vi "Get Next.vi"(0 "Subroutine in":refnum<class "Subroutine.lvclass">, 1 "Linked List Ref":refnum<data-value>, 5 "Active Unique ID":string, 9 "Active Element Index":i32, 11 "error in (no error)":errorcluster) -> (3 "Linked List Ref out":refnum<data-value>, 4 "Executioner out":refnum<class "Executioner.lvclass">, 6 "Active Unique ID out":string, 8 "Test Executive Ref out":refnum<data-value>, 10 "Active Element Index out":i32, 12 "Found":bool, 13 "Complete":bool, 14 "Stop":bool, 15 "error out":errorcluster)   [LabVIEW 2019, in "Test Executive.lvlib" / "Subroutine.lvclass"]
uses:
  <vilib>/gpm_packages/@cs/test-executive/Source/Test Executive/Subroutine/Subroutine.lvclass
  C:/Program Files/National Instruments/LabVIEW 2019/vi.lib/gpm_packages/@cs/test-executive/Source/Test Executive/Executioner/Executioner.lvclass
  <vilib>/gpm_packages/@cs/test-executive/Source/Test Executive/Executioner/Executioner.lvclass
  <vilib>/gpm_packages/@cs/linked-list/Source/Linked List/ILinkedList/ILinked List.lvclass
  <vilib>/gpm_packages/@cs/test-executive/Source/Test Executive/ITestExecutive/ITest Executive.lvclass
  28e86f38-66cc-4303-ad50-260c1a8a0bf4.vi
  bb82cf1c-3602-4c17-aaf6-92fbf2a690c8.vi
  2b196b4b-1a84-4c76-b20a-ced8a0baa885.vi
  296adc96-2638-4d5e-ba7f-24ec80cc44f5.vi
  bf42a184-1053-416f-aa66-ef3d33315e6b.vi
  c3880502-fd26-4328-86fb-66246f65a8d7.vi
  <vilib>/Utility/error.llb/Error Cluster From Error Code.vi
  <vilib>/gpm_packages/@cs/linked-list/Source/Linked List/Linked List Ref/Linked List Ref.lvclass
  <vilib>/gpm_packages/@cs/test-executive/Source/Test Executive/TestExecutive Ref/TestExecutive Ref.lvclass
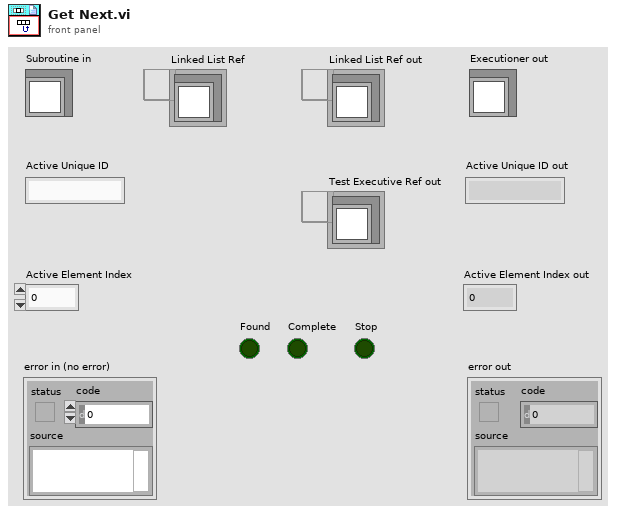
[diagram p1: front panel]
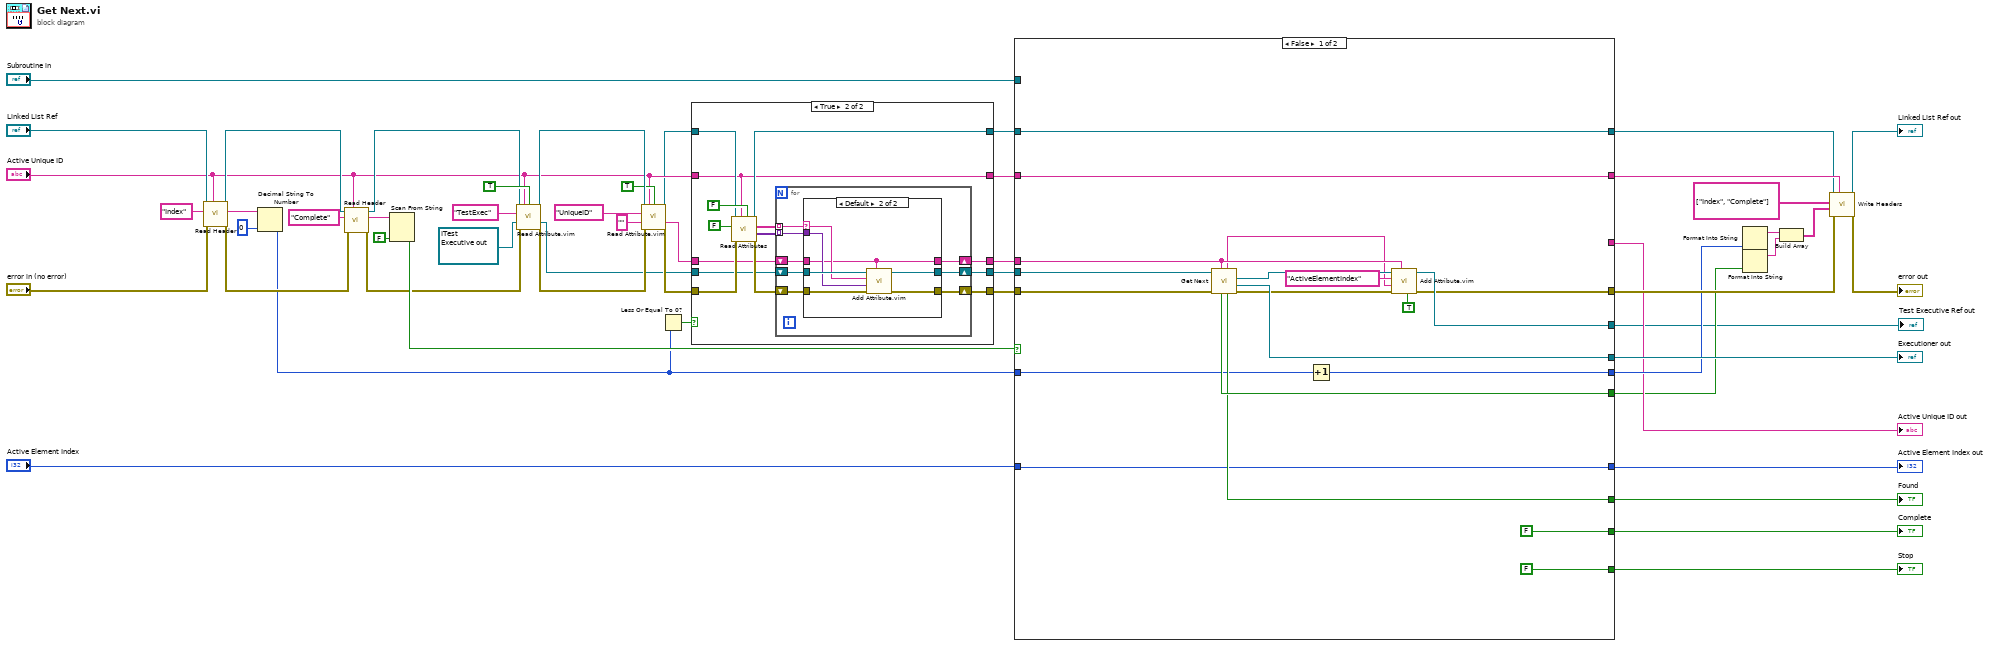
[diagram p0: block diagram]
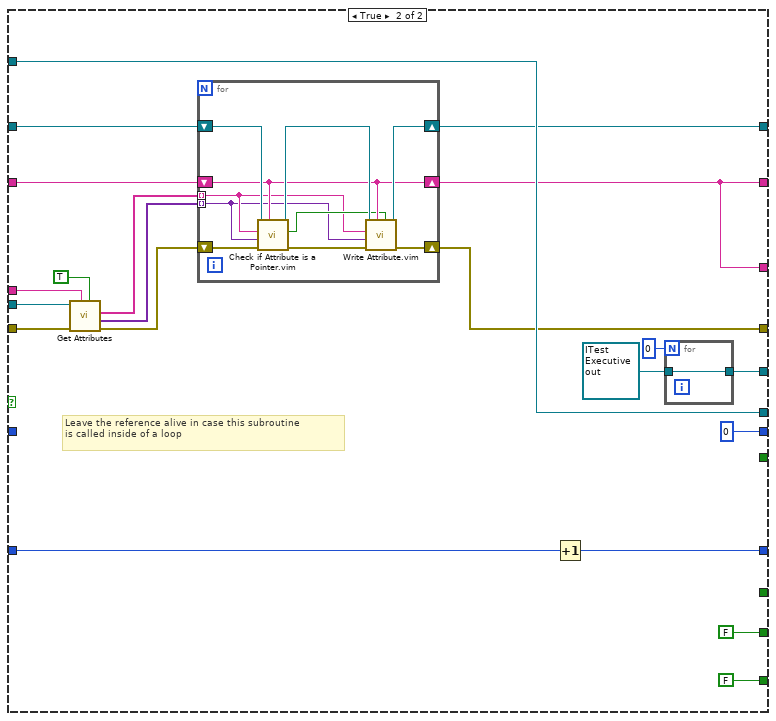
[diagram p4: hidden frame]
diagram:
  n1 = call <vilib>:"Read Header.vi"("Linked List ID"="Active Unique ID", "error in (no error)"="error in (no error)", "Header Name"="Index" ("Attribute Name"), "Linked List Ref"="Linked List Ref") -> ("error out"=w30:errorcluster, "Header Value"=w36:string, "Linked List Ref out"=w31:refnum<data-value>)  [unwired: 4 in, 1 out]
  n2 = Decimal String To Number(string=w36, default (0L)=0 ("Attribute")) -> (number=w1:i32)  [unwired: 1 in, 1 out]
  n3 = call <vilib>:"Read Header.vi"("Linked List ID"="Active Unique ID", "error in (no error)"=w30, "Header Name"="Complete" ("Attribute Name"), "Linked List Ref"=w31) -> ("error out"=w13:errorcluster, "Header Value"=w33:string, "Linked List Ref out"=w14:refnum<data-value>)  [unwired: 4 in, 1 out]
  n4 = Scan From String(input string=w33, default 1=FALSE) -> (output 1=w38:bool)  [unwired: 3 in, 3 out]
  n5 = call "Read Attribute.vim"("Linked List Ref"=w14, "Linked List ID"="Active Unique ID", "Include Private?"=TRUE, "Attribute Name"="TestExec", "Type"=refnum<data-value> refnum ("Test Executive Ref out"), "error in (no error)"=w13) -> ("Linked List Ref out"=w19:refnum<data-value>, "Attribute"=w7:refnum<data-value>, "error out"=w17:errorcluster)  [unwired: 4 in, 3 out]
  n6 = call "Read Attribute.vim"("Linked List Ref"=w19, "Linked List ID"="Active Unique ID", "Include Private?"=TRUE, "Attribute Name"="UniqueID", "Type"="", "error in (no error)"=w17) -> ("Linked List Ref out"=w5:refnum<data-value>, "Attribute"=w9:string, "error out"=w11:errorcluster)  [unwired: 4 in, 3 out]
  n7 = Less Or Equal To 0?(x=w1) -> (x <= 0?=w2:bool)
  n8 = case shown="True" w2 {
    tunnel: "Active Unique ID" -> [w54 w59]
    tunnel: w11 -> [w56 w67]
    tunnel: [w56 w66] -> w10
    tunnel: w9 -> [w55 w65]
    tunnel: [w55 w64] -> w8
    tunnel: w7 -> [w57 w63]
    tunnel: [w57 w62] -> w6
    tunnel: w5 -> [w58 w61]
    tunnel: [w58 w60] -> w4
    tunnel: [w54 w59] -> w3
    frame False {
    }
    frame True {
      n9 = call <vilib>:"Read Attributes.vi"("Flatten Pointer?"=FALSE, "Linked List ID"=w59, "error in (no error)"=w67, "Include Private?"=FALSE, "Linked List Ref"=w61) -> ("error out"=w71:errorcluster, "Attributes"=w68:variant[], "Attribute Names out"=w70:string[], "Linked List Ref out"=w60:refnum<data-value>)  [unwired: 1 in, 2 out]
      n10 = for {
        shift-right: [w77] -> w66
        shift-left: w71 -> [w78]
        tunnel: w70 -> [w76] mode=indexing
        tunnel: w68 -> [w75] mode=indexing
        shift-right: [w74] -> w64
        shift-left: w65 -> [w79]
        shift-right: [w73] -> w62
        shift-left: w63 -> [w80]
        n11 = case shown="Default" w76 {
          selector: w76 -> [_ w87]
          tunnel: w80 -> [w81 w90]
          tunnel: w79 -> [w82 w85]
          tunnel: w78 -> [w83 w89]
          tunnel: [w83 w88] -> w77
          tunnel: w75 -> [_ w86]
          tunnel: [w82 w85] -> w74
          tunnel: [w81 w84] -> w73
          frame "Restore Point" {
          }
          frame Default {
            n12 = call "Add Attribute.vim"("ID"=w85, "error in (no error)"=w89, "Attribute"=w86, "Attribute Name"=w87, "Test Executive Ref"=w90) -> ("error out"=w88:errorcluster, "Test Executive Ref out"=w84:refnum<data-value>)  [unwired: 3 in, 2 out]
          }
        }
      }
    }
  }
  n13 = case shown="False" w38 {
    tunnel: w6 -> [w110 w122]
    tunnel: [w103 w130] -> w48
    tunnel: [w109 _] -> w39
    tunnel: [w100 w116] -> w41
    tunnel: [w108 w118] -> w45
    tunnel: w4 -> [w108 w119]
    tunnel: [w91 0] -> w42
    tunnel: w1 -> [w104 _]
    tunnel: [w107 _] -> w51
    tunnel: [FALSE FALSE] -> w50
    tunnel: [w106 w128] -> w49
    tunnel: "Active Element Index" -> [w106 w131]
    tunnel: "Subroutine in" -> [_ w130]
    tunnel: w10 -> [w105 w121]
    tunnel: [w100 w116] -> w47
    tunnel: w3 -> [w100 w117]
    tunnel: [w96 w111] -> w43
    tunnel: w8 -> [w95 w120]
    tunnel: [w98 w125] -> w24
    tunnel: [FALSE FALSE] -> w23
    frame False {
      n14 = call <vilib>:"Get Next.vi"("Unique ID"=w95, "error in (no error)"=w105, "Test Executive Ref"=w110) -> ("error out"=w97:errorcluster, "Test"=w103:refnum<class "Executioner.lvclass">, "Active Test Executive Ref out"=w99:refnum<data-value>, "Found"=w107:bool, "Unique ID out"=w93:string, "Complete"=w109:bool)  [unwired: 2 in, 1 out]
      n15 = Increment(x=w104) -> (x+1=w91:i32)
      n16 = call "Add Attribute.vim"("Private?"=TRUE, "ID"=w95, "error in (no error)"=w97, "Attribute"=w93, "Attribute Name"="ActiveElementIndex", "Test Executive Ref"=w99) -> ("error out"=w96:errorcluster, "Test Executive Ref out"=w98:refnum<data-value>)  [unwired: 2 in, 2 out]
    }
    frame True {
      # "Leave the reference alive in case this subroutine\nis called inside of a loop"
      n17 = call <vilib>:"Get Attributes.vi"("Flatten Pointer?"=TRUE, "Test ID"=w120, "error in (no error)"=w121, "Test Executive Ref"=w122) -> ("error out"=w113:errorcluster, "Attributes"=w114:variant[], "Attribute Names out"=w115:string[])  [unwired: 2 in, 3 out]
      n18 = for {
        shift-right: [w136] -> w118
        shift-left: w119 -> [w141]
        shift-right: [w135] -> w116
        shift-left: w117 -> [w135]
        tunnel: w115 -> [w133] mode=indexing
        tunnel: w114 -> [w132] mode=indexing
        shift-right: [w138] -> w111
        shift-left: w113 -> [w140]
        n19 = call "Check if Attribute is a Pointer.vim"("Linked List ID"=w135, "error in (no error)"=w140, "Type"=w132, "Attribute Name"=w133, "Linked List Ref"=w141) -> ("error out"=w139:errorcluster, "Pointer?"=w134:bool, "Linked List Ref out"=w137:refnum<data-value>)  [unwired: 2 in, 2 out]
        n20 = call "Write Attribute.vim"("Update Pointer?"=w134, "Linked List ID"=w135, "error in (no error)"=w139, "Attribute"=w132, "Attribute Name"=w133, "Linked List Ref"=w137) -> ("error out"=w138:errorcluster, "Linked List Ref out"=w136:refnum<data-value>)  [unwired: 2 in, 2 out]
      }
      n21 = Increment(x=w131) -> (x+1=w128:i32)
      n22 = for {
        N: 0 -> [_]
        tunnel: refnum<data-value> refnum ("Test Executive Ref out") -> [w142]
        tunnel: [w142] -> w125
      }
    }
  }
  "Executioner out" <- w48
  "Active Unique ID out" <- w41
  "Active Element Index out" <- w49
  "Found" <- w51
  "Complete" <- w50
  "Stop" <- w23
  "Test Executive Ref out" <- w24
  n23 = Format Into String(w42) -> (resulting string=w28:string)  [unwired: 3 in, 1 out]
  n24 = Format Into String(w39) -> (resulting string=w26:string)  [unwired: 3 in, 1 out]
  n25 = Build Array(w28, w26) -> (w27:string[])
  n26 = call <vilib>:"Write Headers.vi"("Linked List ID"=w47, "error in (no error)"=w43, "Header Values"=w27, "Header Names"=string[] ["Index", "Complete"], "Linked List Ref"=w45) -> ("error out"=→"error out":errorcluster, "Linked List Ref out"=→"Linked List Ref out":refnum<data-value>)  [unwired: 5 in]
